vi "UI_visual2.vi"() -> ()   [LabVIEW 2017]
uses:
  <vilib>/Utility/miscctls.llb/LV3DPointTypeDef.ctl
  <vilib>/Analysis/coordinate.llb/Euler Rotation Order.ctl
  <vilib>/picture/3D Picture Control/Object/Create Object (drawable).vi
  <vilib>/picture/3D Picture Control/Object/Create Object (name).vi
  <vilib>/picture/3D Picture Control/Object/Add Object (no reference).vi
  <vilib>/picture/3D Picture Control/Helpers/Apply Texture (no reference).vi
  <vilib>/picture/3D Picture Control/NI_3D Picture Control.lvlib
  <vilib>/Analysis/NI_AALPro.lvlib
  <vilib>/picture/3D Picture Control/Helpers/Set Clip Plane (no reference).vi
panel:
  out "V_ini [m/s]":dbl[][](array[numeric])
  out "Euler Angles [rad]":dbl[](array[numeric])
  in  "Sim_Time":dbl=40.0
  in  "Tab Control":T1(tab)
  out "Position":dbl[][](graph)
  out "Velocity [m/s]":cluster{dbl, dbl, "V_ini [m/s]":dbl[]}(graph)
  out "Quaternions":dbl[][](graph)
  out "Euler Angles [º]":cluster{dbl, dbl, dbl[][]}(graph)
  out "Body Rates":dbl[][](graph)
  out "Body accelerations":dbl[][](graph)
  out "Malpha/Mbeta":dbl[][](graph)
  out "AoA":dbl[][](graph)
  out "TVA angles":dbl[][](graph)
  out "Oil Consumption":dbl[][](graph)
  out "Bending Moments":dbl[][](graph)
  out "Aerodynamic pressure":dbl[](graph)
  out "Sim_Stopped":bool
  in  "stop Host":bool
  in  "Run_SIM":bool
  out "time[s]":dbl
  out "Euler Angles [º]":dbl[](array[numeric])
  out "B-frame [m]":cluster{"X":sgl, "Y":sgl, "Z":sgl}
  in  "B-frame Translation 2":cluster{"X":sgl, "Y":sgl, "Z":sgl}
  in  "N-frame rot":dbl[](array[numeric])
  in  "Up Direction":T2={"X"=0.0, "Y"=0.0, "Z"=1.0}
  out "3D Picture Control":refnum<vi>(3d-picture)
  in  "error in (no error)":errorcluster
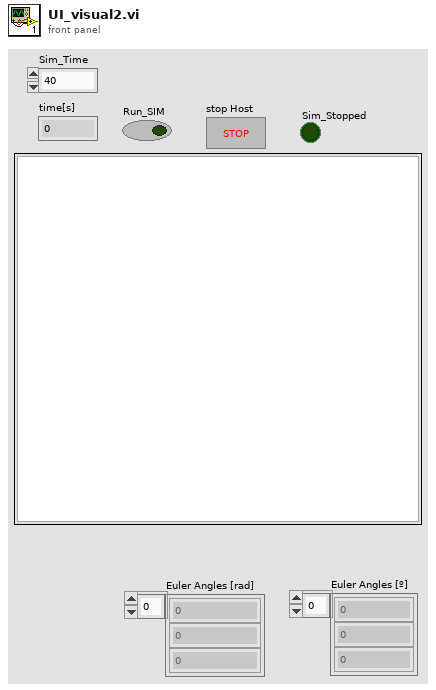
[diagram p1: front panel]
types:
  T1 = enum32{"Position", "Velocity", "Attitude Quaternions", "Attitude Euler Angles", "Body Rates", "Body Accel", "Malpha/ Mbeta", "AoA", "TVA nozzle angles", "Oil Consumption", "Bending Moments", "Aerodynamic pressure"}
  T2 = typedef "LV3DPointTypeDef.ctl" = cluster{"X":sgl, "Y":sgl, "Z":sgl}
  T3 = enum16{"As a Decal", "With Modulation", "With Blending", "As a replacement"}
  T4 = cluster{"Red":sgl, "Green":sgl, "Blue":sgl, "Alpha":sgl}
  T5 = typedef "NI_AALPro.lvlib/Euler Rotation Order.ctl" = u16
  T6 = typedef "imagedata.ctl" = cluster{"image type":i32, "image depth":i32, "image":u8[], "mask":u8[], "colors":u32[], "Rectangle":cluster{"left":i16, "top":i16, "right":i16, "bottom":i16}}
  T7 = cluster{"element":dbl, "element":dbl, "element":dbl}
  T8 = cluster{dbl, "latd_ini [º]":dbl, "lon_ini [º]":dbl, "alt_ini(m)":dbl, "V_ini [m/s]":dbl[], "q ini":dbl[], dbl[], "W ini [rad/s]":dbl[], "acc":dbl[], dbl[], dbl[], "TVA_b":dbl[], "array":dbl[], "array":dbl[], "Pdin":dbl}
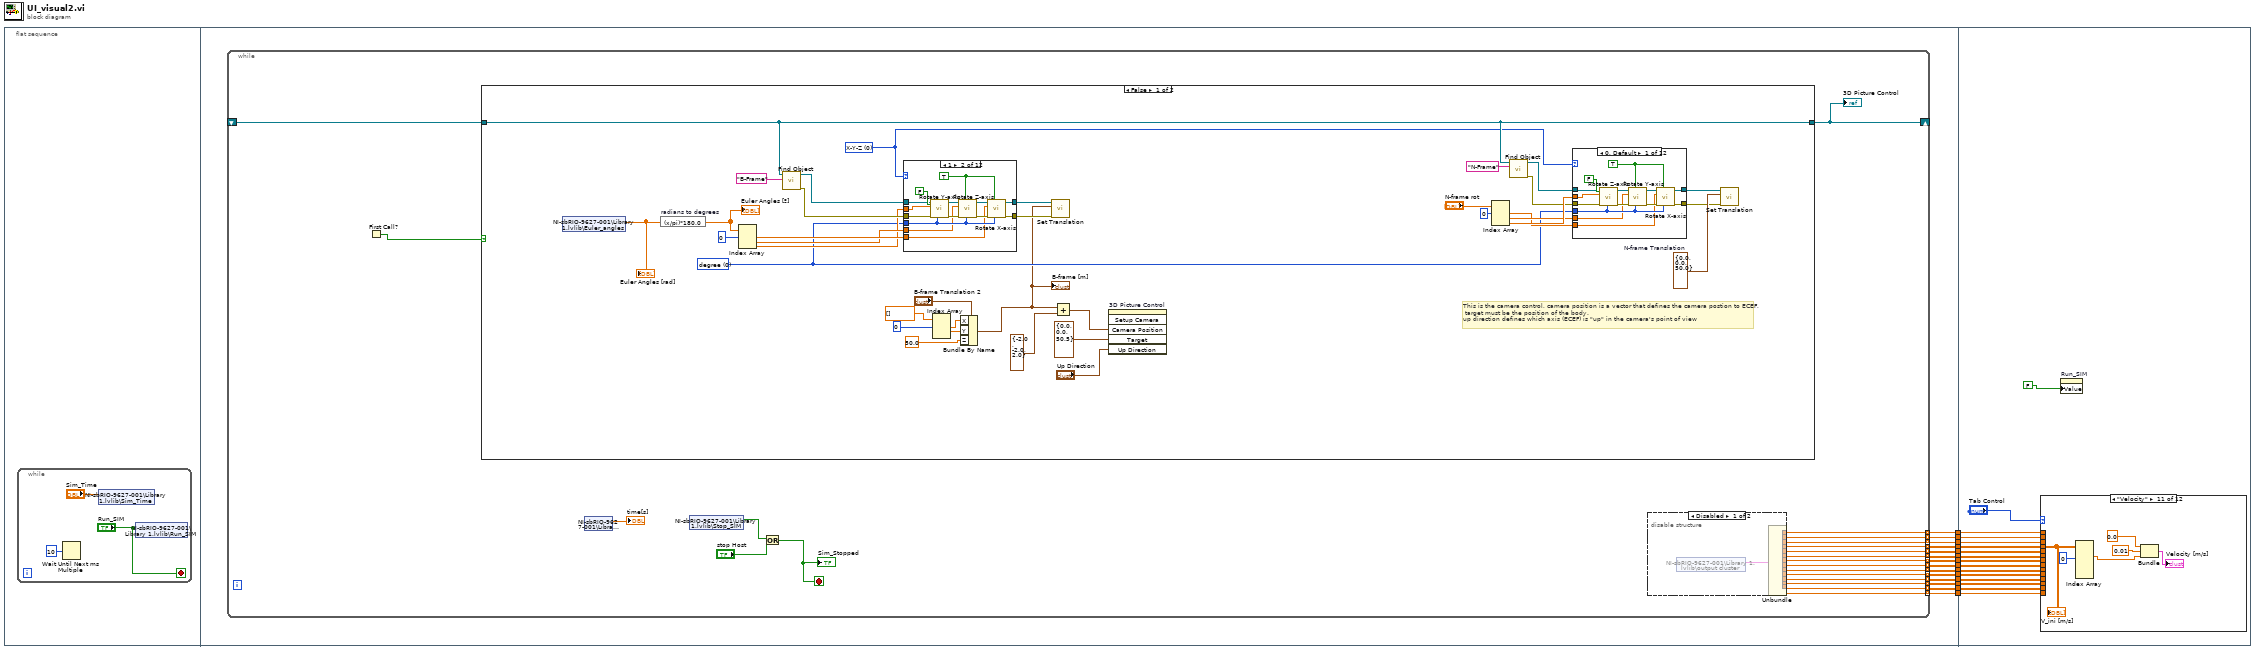
[diagram p0: block diagram]
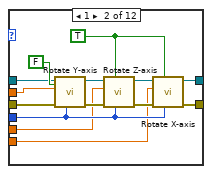
[diagram p3: hidden frame]
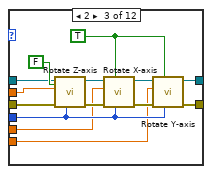
[diagram p4: hidden frame]
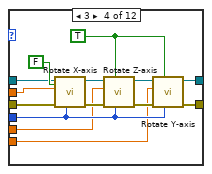
[diagram p5: hidden frame]
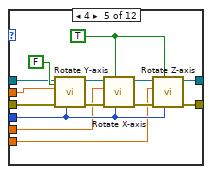
[diagram p6: hidden frame]
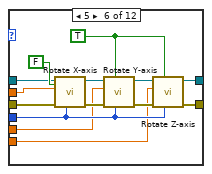
[diagram p7: hidden frame]
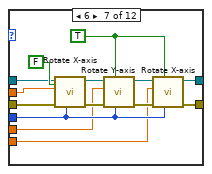
[diagram p8: hidden frame]
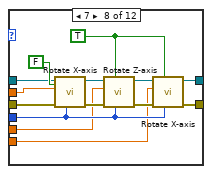
[diagram p9: hidden frame]
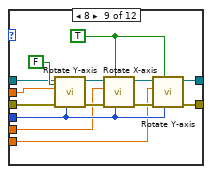
[diagram p10: hidden frame]
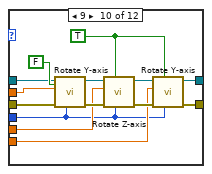
[diagram p11: hidden frame]
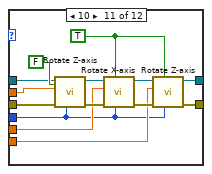
[diagram p12: hidden frame]
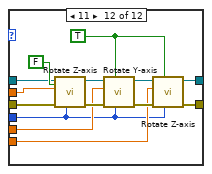
[diagram p13: hidden frame]
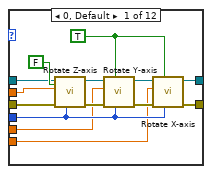
[diagram p14: hidden frame]
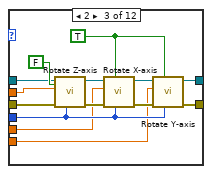
[diagram p15: hidden frame]
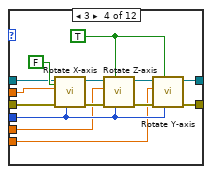
[diagram p16: hidden frame]
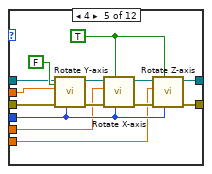
[diagram p17: hidden frame]
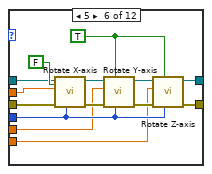
[diagram p18: hidden frame]
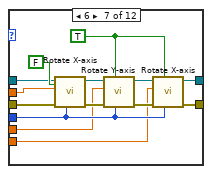
[diagram p19: hidden frame]
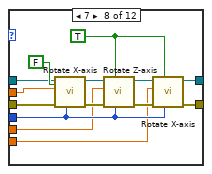
[diagram p20: hidden frame]
diagram:
  n1 = flat-sequence {
    tunnel: [w31] -> w14
    tunnel: [w30] -> w13
    tunnel: [w29] -> w12
    tunnel: [w28] -> w11
    tunnel: [w27] -> w10
    tunnel: [w26] -> w9
    tunnel: [w25] -> w8
    tunnel: [w24] -> w7
    tunnel: [w23] -> w6
    tunnel: [w22] -> w5
    tunnel: [w21] -> w4
    tunnel: [w20] -> w3
    tunnel: [w19] -> w2
    tunnel: [w18] -> w1
    tunnel: w14 -> [w533]
    tunnel: w13 -> [w532]
    tunnel: w12 -> [w531]
    tunnel: w11 -> [w530]
    tunnel: w10 -> [w529]
    tunnel: w9 -> [w528]
    tunnel: w8 -> [w527]
    tunnel: w7 -> [w526]
    tunnel: w6 -> [w525]
    tunnel: w5 -> [w524]
    tunnel: w4 -> [w523]
    tunnel: w3 -> [w522]
    tunnel: w2 -> [w521]
    tunnel: w1 -> [w520]
    frame #0 {
      n2 = while {
        stop <- "Run_SIM" stop-if-true
        n3 = Wait Until Next ms Multiple(millisecond multiple=u32 10) -> ()  [unwired: 1 out]
        n4 = shared-variable "NI-sbRIO-9627-001\\Library 1.lvlib\\Sim_Time"("Sim_Time") -> ()  [unwired: 1 in, 1 out]
        n5 = shared-variable "NI-sbRIO-9627-001\\Library 1.lvlib\\Run_SIM"("Run_SIM") -> ()  [unwired: 1 in, 1 out]
      }
    }
    frame #1 {
      n6 = while {
        shift-right: [w51] -> _
        shift-left: _ -> [w52]
        tunnel: [w45] -> w31 mode=indexing
        tunnel: [w44] -> w30 mode=indexing
        tunnel: [w43] -> w29 mode=indexing
        tunnel: [w42] -> w28 mode=indexing
        tunnel: [w41] -> w27 mode=indexing
        tunnel: [w40] -> w26 mode=indexing
        tunnel: [w39] -> w25 mode=indexing
        tunnel: [w38] -> w24 mode=indexing
        tunnel: [w37] -> w23 mode=indexing
        tunnel: [w36] -> w22 mode=indexing
        tunnel: [w35] -> w21 mode=indexing
        tunnel: [w34] -> w20 mode=indexing
        tunnel: [w33] -> w19 mode=indexing
        tunnel: [w32] -> w18 mode=indexing
        stop <- w48 stop-if-true
        n7 = First Call?() -> (First Call?: T/F=w50:bool)
        n8 = case shown="False" w50 {
          tunnel: [w84 w447] -> w51
          tunnel: w52 -> [w84 _]
          frame False {
            w83 = T5 0 items=["X-Y-Z", "X-Z-Y", "Y-X-Z", "Y-Z-X", "Z-X-Y", "Z-Y-X", "X-Y-X", "X-Z-X", "Y-X-Y", "Y-Z-Y", "Z-X-Z", "Z-Y-Z"] ("rotation order")
            w94 = cluster{"X":sgl, "Y":sgl, "Z":sgl} {"X"=0.0, "Y"=0.0, "Z"=50.0}  # N-frame Translation
            w82 = u16 0 items=["degree", "radians"] ("angle unit")
            # "This is the camera control, camera position is a vector that defines the camera postion to ECEF,\n target must be the position of the body. \nup direction defines which axis (ECEF) is \"up\" in the camera's point of view"
            n9 = shared-variable "NI-sbRIO-9627-001\\Library 1.lvlib\\Euler_angles"() -> (w76:dbl[])  [unwired: 1 in, 1 out]
            "Euler Angles [rad]" <- w76
            n10 = expression code="(x/pi)*180.0" "radians to degrees"(w76) -> (w77:dbl[])
            "Euler Angles [º]" <- w77
            n11 = Index Array(array=w77, index #1=0 ("index")) -> (element #1=w102:dbl, element #2=w99:dbl, element #3=w98:dbl)  [unwired: 2 in]
            n12 = call <vilib>:"Find Object.vi"("Object Name"="B-Frame", "Scene Refnum"=w84) -> ("error out"=w100:errorcluster, "Object Refnum"=w101:refnum<vi>)  [unwired: 8 in]
            n13 = case shown="1" w83 {
              tunnel: w102 -> [w276 w292 w306 w320 w330 w348 w362 w376 w390 w401 w415 w429]
              tunnel: w101 -> [w279 w289 w302 w316 w334 w344 w361 w375 w386 w405 w419 w433]
              tunnel: w100 -> [w278 w288 w303 w317 w333 w345 w360 w374 w387 w404 w418 w432]
              tunnel: w99 -> [w275 w290 w305 w319 w331 w347 w358 w372 w389 w402 w416 w431]
              tunnel: w98 -> [w274 w291 w304 w318 w332 w346 w359 w373 w388 w403 w417 w430]
              tunnel: w82 -> [w277 w293 w307 w321 w335 w349 w363 w377 w391 w400 w414 w428]
              tunnel: [w273 w287 w301 w315 w329 w343 w357 w371 w385 w399 w413 w427] -> w96
              tunnel: [w272 w286 w300 w314 w328 w342 w356 w370 w384 w398 w412 w426] -> w95
              frame 0, Default {
                w285 = TRUE ("Relative?")
                n14 = call <vilib>:"Rotate Z-axis.vi"("angle unit"=w277, "Relative?"=FALSE, "error in (no error)"=w278, "angle"=w274, "Scene Object In"=w279) -> ("error out"=w282:errorcluster, "Scene Object Out"=w283:refnum<vi>)  [unwired: 5 in]
                n15 = call <vilib>:"Rotate Y-axis.vi"("angle unit"=w277, "Relative?"=w285, "error in (no error)"=w282, "angle"=w275, "Scene Object In"=w283) -> ("error out"=w281:errorcluster, "Scene Object Out"=w280:refnum<vi>)  [unwired: 5 in]
                n16 = call <vilib>:"Rotate X-axis.vi"("angle unit"=w277, "Relative?"=w285, "error in (no error)"=w281, "angle"=w276, "Scene Object In"=w280) -> ("error out"=w272:errorcluster, "Scene Object Out"=w273:refnum<vi>)  [unwired: 5 in]
              }
              frame 1 {
                w296 = TRUE ("Relative?")
                n17 = call <vilib>:"Rotate Y-axis.vi"("angle unit"=w293, "Relative?"=FALSE, "error in (no error)"=w288, "angle"=w291, "Scene Object In"=w289) -> ("error out"=w297:errorcluster, "Scene Object Out"=w298:refnum<vi>)  [unwired: 5 in]
                n18 = call <vilib>:"Rotate Z-axis.vi"("angle unit"=w293, "Relative?"=w296, "error in (no error)"=w297, "angle"=w290, "Scene Object In"=w298) -> ("error out"=w294:errorcluster, "Scene Object Out"=w295:refnum<vi>)  [unwired: 5 in]
                n19 = call <vilib>:"Rotate X-axis.vi"("angle unit"=w293, "Relative?"=w296, "error in (no error)"=w294, "angle"=w292, "Scene Object In"=w295) -> ("error out"=w286:errorcluster, "Scene Object Out"=w287:refnum<vi>)  [unwired: 5 in]
              }
              frame 2 {
                w308 = TRUE ("Relative?")
                n20 = call <vilib>:"Rotate Z-axis.vi"("angle unit"=w307, "Relative?"=FALSE, "error in (no error)"=w303, "angle"=w304, "Scene Object In"=w302) -> ("error out"=w311:errorcluster, "Scene Object Out"=w312:refnum<vi>)  [unwired: 5 in]
                n21 = call <vilib>:"Rotate X-axis.vi"("angle unit"=w307, "Relative?"=w308, "error in (no error)"=w311, "angle"=w305, "Scene Object In"=w312) -> ("error out"=w309:errorcluster, "Scene Object Out"=w310:refnum<vi>)  [unwired: 5 in]
                n22 = call <vilib>:"Rotate Y-axis.vi"("angle unit"=w307, "Relative?"=w308, "error in (no error)"=w309, "angle"=w306, "Scene Object In"=w310) -> ("error out"=w300:errorcluster, "Scene Object Out"=w301:refnum<vi>)  [unwired: 5 in]
              }
              frame 3 {
                w326 = TRUE ("Relative?")
                n23 = call <vilib>:"Rotate X-axis.vi"("angle unit"=w321, "Relative?"=FALSE, "error in (no error)"=w317, "angle"=w318, "Scene Object In"=w316) -> ("error out"=w324:errorcluster, "Scene Object Out"=w325:refnum<vi>)  [unwired: 5 in]
                n24 = call <vilib>:"Rotate Z-axis.vi"("angle unit"=w321, "Relative?"=w326, "error in (no error)"=w324, "angle"=w319, "Scene Object In"=w325) -> ("error out"=w322:errorcluster, "Scene Object Out"=w323:refnum<vi>)  [unwired: 5 in]
                n25 = call <vilib>:"Rotate Y-axis.vi"("angle unit"=w321, "Relative?"=w326, "error in (no error)"=w322, "angle"=w320, "Scene Object In"=w323) -> ("error out"=w314:errorcluster, "Scene Object Out"=w315:refnum<vi>)  [unwired: 5 in]
              }
              frame 4 {
                w340 = TRUE ("Relative?")
                n26 = call <vilib>:"Rotate Y-axis.vi"("angle unit"=w335, "Relative?"=FALSE, "error in (no error)"=w333, "angle"=w332, "Scene Object In"=w334) -> ("error out"=w336:errorcluster, "Scene Object Out"=w337:refnum<vi>)  [unwired: 5 in]
                n27 = call <vilib>:"Rotate X-axis.vi"("angle unit"=w335, "Relative?"=w340, "error in (no error)"=w336, "angle"=w331, "Scene Object In"=w337) -> ("error out"=w339:errorcluster, "Scene Object Out"=w338:refnum<vi>)  [unwired: 5 in]
                n28 = call <vilib>:"Rotate Z-axis.vi"("angle unit"=w335, "Relative?"=w340, "error in (no error)"=w339, "angle"=w330, "Scene Object In"=w338) -> ("error out"=w328:errorcluster, "Scene Object Out"=w329:refnum<vi>)  [unwired: 5 in]
              }
              frame 5 {
                w353 = TRUE ("Relative?")
                n29 = call <vilib>:"Rotate X-axis.vi"("angle unit"=w349, "Relative?"=FALSE, "error in (no error)"=w345, "angle"=w346, "Scene Object In"=w344) -> ("error out"=w351:errorcluster, "Scene Object Out"=w352:refnum<vi>)  [unwired: 5 in]
                n30 = call <vilib>:"Rotate Y-axis.vi"("angle unit"=w349, "Relative?"=w353, "error in (no error)"=w351, "angle"=w347, "Scene Object In"=w352) -> ("error out"=w355:errorcluster, "Scene Object Out"=w354:refnum<vi>)  [unwired: 5 in]
                n31 = call <vilib>:"Rotate Z-axis.vi"("angle unit"=w349, "Relative?"=w353, "error in (no error)"=w355, "angle"=w348, "Scene Object In"=w354) -> ("error out"=w342:errorcluster, "Scene Object Out"=w343:refnum<vi>)  [unwired: 5 in]
              }
              frame 6 {
                w366 = TRUE ("Relative?")
                n32 = call <vilib>:"Rotate X-axis.vi"("angle unit"=w363, "Relative?"=FALSE, "error in (no error)"=w360, "angle"=w359, "Scene Object In"=w361) -> ("error out"=w368:errorcluster, "Scene Object Out"=w369:refnum<vi>)  [unwired: 5 in]
                n33 = call <vilib>:"Rotate Y-axis.vi"("angle unit"=w363, "Relative?"=w366, "error in (no error)"=w368, "angle"=w358, "Scene Object In"=w369) -> ("error out"=w364:errorcluster, "Scene Object Out"=w365:refnum<vi>)  [unwired: 5 in]
                n34 = call <vilib>:"Rotate X-axis.vi"("angle unit"=w363, "Relative?"=w366, "error in (no error)"=w364, "angle"=w362, "Scene Object In"=w365) -> ("error out"=w356:errorcluster, "Scene Object Out"=w357:refnum<vi>)  [unwired: 5 in]
              }
              frame 7 {
                w382 = TRUE ("Relative?")
                n35 = call <vilib>:"Rotate X-axis.vi"("angle unit"=w377, "Relative?"=FALSE, "error in (no error)"=w374, "angle"=w373, "Scene Object In"=w375) -> ("error out"=w380:errorcluster, "Scene Object Out"=w381:refnum<vi>)  [unwired: 5 in]
                n36 = call <vilib>:"Rotate Z-axis.vi"("angle unit"=w377, "Relative?"=w382, "error in (no error)"=w380, "angle"=w372, "Scene Object In"=w381) -> ("error out"=w379:errorcluster, "Scene Object Out"=w378:refnum<vi>)  [unwired: 5 in]
                n37 = call <vilib>:"Rotate X-axis.vi"("angle unit"=w377, "Relative?"=w382, "error in (no error)"=w379, "angle"=w376, "Scene Object In"=w378) -> ("error out"=w370:errorcluster, "Scene Object Out"=w371:refnum<vi>)  [unwired: 5 in]
              }
              frame 8 {
                w396 = TRUE ("Relative?")
                n38 = call <vilib>:"Rotate Y-axis.vi"("angle unit"=w391, "Relative?"=FALSE, "error in (no error)"=w387, "angle"=w388, "Scene Object In"=w386) -> ("error out"=w394:errorcluster, "Scene Object Out"=w395:refnum<vi>)  [unwired: 5 in]
                n39 = call <vilib>:"Rotate X-axis.vi"("angle unit"=w391, "Relative?"=w396, "error in (no error)"=w394, "angle"=w389, "Scene Object In"=w395) -> ("error out"=w393:errorcluster, "Scene Object Out"=w392:refnum<vi>)  [unwired: 5 in]
                n40 = call <vilib>:"Rotate Y-axis.vi"("angle unit"=w391, "Relative?"=w396, "error in (no error)"=w393, "angle"=w390, "Scene Object In"=w392) -> ("error out"=w384:errorcluster, "Scene Object Out"=w385:refnum<vi>)  [unwired: 5 in]
              }
              frame 9 {
                w410 = TRUE ("Relative?")
                n41 = call <vilib>:"Rotate Y-axis.vi"("angle unit"=w400, "Relative?"=FALSE, "error in (no error)"=w404, "angle"=w403, "Scene Object In"=w405) -> ("error out"=w408:errorcluster, "Scene Object Out"=w409:refnum<vi>)  [unwired: 5 in]
                n42 = call <vilib>:"Rotate Z-axis.vi"("angle unit"=w400, "Relative?"=w410, "error in (no error)"=w408, "angle"=w402, "Scene Object In"=w409) -> ("error out"=w407:errorcluster, "Scene Object Out"=w406:refnum<vi>)  [unwired: 5 in]
                n43 = call <vilib>:"Rotate Y-axis.vi"("angle unit"=w400, "Relative?"=w410, "error in (no error)"=w407, "angle"=w401, "Scene Object In"=w406) -> ("error out"=w398:errorcluster, "Scene Object Out"=w399:refnum<vi>)  [unwired: 5 in]
              }
              frame 10 {
                w424 = TRUE ("Relative?")
                n44 = call <vilib>:"Rotate Z-axis.vi"("angle unit"=w414, "Relative?"=FALSE, "error in (no error)"=w418, "angle"=w417, "Scene Object In"=w419) -> ("error out"=w422:errorcluster, "Scene Object Out"=w423:refnum<vi>)  [unwired: 5 in]
                n45 = call <vilib>:"Rotate X-axis.vi"("angle unit"=w414, "Relative?"=w424, "error in (no error)"=w422, "angle"=w416, "Scene Object In"=w423) -> ("error out"=w421:errorcluster, "Scene Object Out"=w420:refnum<vi>)  [unwired: 5 in]
                n46 = call <vilib>:"Rotate Z-axis.vi"("angle unit"=w414, "Relative?"=w424, "error in (no error)"=w421, "angle"=w415, "Scene Object In"=w420) -> ("error out"=w412:errorcluster, "Scene Object Out"=w413:refnum<vi>)  [unwired: 5 in]
              }
              frame 11 {
                w438 = TRUE ("Relative?")
                n47 = call <vilib>:"Rotate Z-axis.vi"("angle unit"=w428, "Relative?"=FALSE, "error in (no error)"=w432, "angle"=w430, "Scene Object In"=w433) -> ("error out"=w436:errorcluster, "Scene Object Out"=w437:refnum<vi>)  [unwired: 5 in]
                n48 = call <vilib>:"Rotate Y-axis.vi"("angle unit"=w428, "Relative?"=w438, "error in (no error)"=w436, "angle"=w431, "Scene Object In"=w437) -> ("error out"=w435:errorcluster, "Scene Object Out"=w434:refnum<vi>)  [unwired: 5 in]
                n49 = call <vilib>:"Rotate Z-axis.vi"("angle unit"=w428, "Relative?"=w438, "error in (no error)"=w435, "angle"=w429, "Scene Object In"=w434) -> ("error out"=w426:errorcluster, "Scene Object Out"=w427:refnum<vi>)  [unwired: 5 in]
              }
            }
            n50 = Index Array(array=dbl[] [], index #1=0 ("index")) -> (element #1=w79:dbl, element #2=w78:dbl)  [unwired: 2 in, 1 out]
            n51 = Bundle By Name(cluster="B-frame Translation 2", "X"=w79, "Y"=w78, "Z"=50.0 ("Double")) -> (w70:cluster{"X":sgl, "Y":sgl, "Z":sgl})
            "B-frame [m]" <- w70
            n52 = call <vilib>:"Set Translation.vi"("error in (no error)"=w95, "Translation"=w70, "Scene Object"=w96) -> ()  [unwired: 7 in, 2 out]
            n53 = Add(x=w70, y=T2 {"X"=-2.0, "Y"=-2.0, "Z"=2.0} ("Camera Position control")) -> (x+y=w71:T2)
            n54 = invoke on="3D Picture Control" class="SceneGraphDisp (strict)" method="Setup Camera"("Camera Position"=w71, "Target"=T2 {"X"=0.0, "Y"=0.0, "Z"=50.5}, "Up Direction"="Up Direction") -> ()  [unwired: 3 in, 6 out]
            n55 = Index Array(array="N-frame rot", index #1=0 ("index")) -> (element #1=w86:dbl, element #2=w89:dbl, element #3=w90:dbl)  [unwired: 2 in]
            n56 = call <vilib>:"Find Object.vi"("Object Name"="N-Frame", "Scene Refnum"=w84) -> ("error out"=w88:errorcluster, "Object Refnum"=w87:refnum<vi>)  [unwired: 8 in]
            n57 = case shown="0, Default" w83 {
              tunnel: w86 -> [w108 w124 w138 w152 w162 w180 w194 w208 w222 w233 w247 w261]
              tunnel: w87 -> [w111 w121 w134 w148 w166 w176 w193 w207 w218 w237 w251 w265]
              tunnel: w88 -> [w110 w120 w135 w149 w165 w177 w192 w206 w219 w236 w250 w264]
              tunnel: w89 -> [w107 w122 w137 w151 w163 w179 w190 w204 w221 w234 w248 w263]
              tunnel: w90 -> [w106 w123 w136 w150 w164 w178 w191 w205 w220 w235 w249 w262]
              tunnel: w82 -> [w109 w125 w139 w153 w167 w181 w195 w209 w223 w232 w246 w260]
              tunnel: [w105 w119 w133 w147 w161 w175 w189 w203 w217 w231 w245 w259] -> w92
              tunnel: [w104 w118 w132 w146 w160 w174 w188 w202 w216 w230 w244 w258] -> w93
              frame 0, Default {
                w117 = TRUE ("Relative?")
                n58 = call <vilib>:"Rotate Z-axis.vi"("angle unit"=w109, "Relative?"=FALSE, "error in (no error)"=w110, "angle"=w106, "Scene Object In"=w111) -> ("error out"=w114:errorcluster, "Scene Object Out"=w115:refnum<vi>)  [unwired: 5 in]
                n59 = call <vilib>:"Rotate Y-axis.vi"("angle unit"=w109, "Relative?"=w117, "error in (no error)"=w114, "angle"=w107, "Scene Object In"=w115) -> ("error out"=w113:errorcluster, "Scene Object Out"=w112:refnum<vi>)  [unwired: 5 in]
                n60 = call <vilib>:"Rotate X-axis.vi"("angle unit"=w109, "Relative?"=w117, "error in (no error)"=w113, "angle"=w108, "Scene Object In"=w112) -> ("error out"=w104:errorcluster, "Scene Object Out"=w105:refnum<vi>)  [unwired: 5 in]
              }
              frame 1 {
                w128 = TRUE ("Relative?")
                n61 = call <vilib>:"Rotate Y-axis.vi"("angle unit"=w125, "Relative?"=FALSE, "error in (no error)"=w120, "angle"=w123, "Scene Object In"=w121) -> ("error out"=w129:errorcluster, "Scene Object Out"=w130:refnum<vi>)  [unwired: 5 in]
                n62 = call <vilib>:"Rotate Z-axis.vi"("angle unit"=w125, "Relative?"=w128, "error in (no error)"=w129, "angle"=w122, "Scene Object In"=w130) -> ("error out"=w126:errorcluster, "Scene Object Out"=w127:refnum<vi>)  [unwired: 5 in]
                n63 = call <vilib>:"Rotate X-axis.vi"("angle unit"=w125, "Relative?"=w128, "error in (no error)"=w126, "angle"=w124, "Scene Object In"=w127) -> ("error out"=w118:errorcluster, "Scene Object Out"=w119:refnum<vi>)  [unwired: 5 in]
              }
              frame 2 {
                w140 = TRUE ("Relative?")
                n64 = call <vilib>:"Rotate Z-axis.vi"("angle unit"=w139, "Relative?"=FALSE, "error in (no error)"=w135, "angle"=w136, "Scene Object In"=w134) -> ("error out"=w143:errorcluster, "Scene Object Out"=w144:refnum<vi>)  [unwired: 5 in]
                n65 = call <vilib>:"Rotate X-axis.vi"("angle unit"=w139, "Relative?"=w140, "error in (no error)"=w143, "angle"=w137, "Scene Object In"=w144) -> ("error out"=w141:errorcluster, "Scene Object Out"=w142:refnum<vi>)  [unwired: 5 in]
                n66 = call <vilib>:"Rotate Y-axis.vi"("angle unit"=w139, "Relative?"=w140, "error in (no error)"=w141, "angle"=w138, "Scene Object In"=w142) -> ("error out"=w132:errorcluster, "Scene Object Out"=w133:refnum<vi>)  [unwired: 5 in]
              }
              frame 3 {
                w158 = TRUE ("Relative?")
                n67 = call <vilib>:"Rotate X-axis.vi"("angle unit"=w153, "Relative?"=FALSE, "error in (no error)"=w149, "angle"=w150, "Scene Object In"=w148) -> ("error out"=w156:errorcluster, "Scene Object Out"=w157:refnum<vi>)  [unwired: 5 in]
                n68 = call <vilib>:"Rotate Z-axis.vi"("angle unit"=w153, "Relative?"=w158, "error in (no error)"=w156, "angle"=w151, "Scene Object In"=w157) -> ("error out"=w154:errorcluster, "Scene Object Out"=w155:refnum<vi>)  [unwired: 5 in]
                n69 = call <vilib>:"Rotate Y-axis.vi"("angle unit"=w153, "Relative?"=w158, "error in (no error)"=w154, "angle"=w152, "Scene Object In"=w155) -> ("error out"=w146:errorcluster, "Scene Object Out"=w147:refnum<vi>)  [unwired: 5 in]
              }
              frame 4 {
                w172 = TRUE ("Relative?")
                n70 = call <vilib>:"Rotate Y-axis.vi"("angle unit"=w167, "Relative?"=FALSE, "error in (no error)"=w165, "angle"=w164, "Scene Object In"=w166) -> ("error out"=w168:errorcluster, "Scene Object Out"=w169:refnum<vi>)  [unwired: 5 in]
                n71 = call <vilib>:"Rotate X-axis.vi"("angle unit"=w167, "Relative?"=w172, "error in (no error)"=w168, "angle"=w163, "Scene Object In"=w169) -> ("error out"=w171:errorcluster, "Scene Object Out"=w170:refnum<vi>)  [unwired: 5 in]
                n72 = call <vilib>:"Rotate Z-axis.vi"("angle unit"=w167, "Relative?"=w172, "error in (no error)"=w171, "angle"=w162, "Scene Object In"=w170) -> ("error out"=w160:errorcluster, "Scene Object Out"=w161:refnum<vi>)  [unwired: 5 in]
              }
              frame 5 {
                w185 = TRUE ("Relative?")
                n73 = call <vilib>:"Rotate X-axis.vi"("angle unit"=w181, "Relative?"=FALSE, "error in (no error)"=w177, "angle"=w178, "Scene Object In"=w176) -> ("error out"=w183:errorcluster, "Scene Object Out"=w184:refnum<vi>)  [unwired: 5 in]
                n74 = call <vilib>:"Rotate Y-axis.vi"("angle unit"=w181, "Relative?"=w185, "error in (no error)"=w183, "angle"=w179, "Scene Object In"=w184) -> ("error out"=w187:errorcluster, "Scene Object Out"=w186:refnum<vi>)  [unwired: 5 in]
                n75 = call <vilib>:"Rotate Z-axis.vi"("angle unit"=w181, "Relative?"=w185, "error in (no error)"=w187, "angle"=w180, "Scene Object In"=w186) -> ("error out"=w174:errorcluster, "Scene Object Out"=w175:refnum<vi>)  [unwired: 5 in]
              }
              frame 6 {
                w198 = TRUE ("Relative?")
                n76 = call <vilib>:"Rotate X-axis.vi"("angle unit"=w195, "Relative?"=FALSE, "error in (no error)"=w192, "angle"=w191, "Scene Object In"=w193) -> ("error out"=w200:errorcluster, "Scene Object Out"=w201:refnum<vi>)  [unwired: 5 in]
                n77 = call <vilib>:"Rotate Y-axis.vi"("angle unit"=w195, "Relative?"=w198, "error in (no error)"=w200, "angle"=w190, "Scene Object In"=w201) -> ("error out"=w196:errorcluster, "Scene Object Out"=w197:refnum<vi>)  [unwired: 5 in]
                n78 = call <vilib>:"Rotate X-axis.vi"("angle unit"=w195, "Relative?"=w198, "error in (no error)"=w196, "angle"=w194, "Scene Object In"=w197) -> ("error out"=w188:errorcluster, "Scene Object Out"=w189:refnum<vi>)  [unwired: 5 in]
              }
              frame 7 {
                w214 = TRUE ("Relative?")
                n79 = call <vilib>:"Rotate X-axis.vi"("angle unit"=w209, "Relative?"=FALSE, "error in (no error)"=w206, "angle"=w205, "Scene Object In"=w207) -> ("error out"=w212:errorcluster, "Scene Object Out"=w213:refnum<vi>)  [unwired: 5 in]
                n80 = call <vilib>:"Rotate Z-axis.vi"("angle unit"=w209, "Relative?"=w214, "error in (no error)"=w212, "angle"=w204, "Scene Object In"=w213) -> ("error out"=w211:errorcluster, "Scene Object Out"=w210:refnum<vi>)  [unwired: 5 in]
                n81 = call <vilib>:"Rotate X-axis.vi"("angle unit"=w209, "Relative?"=w214, "error in (no error)"=w211, "angle"=w208, "Scene Object In"=w210) -> ("error out"=w202:errorcluster, "Scene Object Out"=w203:refnum<vi>)  [unwired: 5 in]
              }
              frame 8 {
                w228 = TRUE ("Relative?")
                n82 = call <vilib>:"Rotate Y-axis.vi"("angle unit"=w223, "Relative?"=FALSE, "error in (no error)"=w219, "angle"=w220, "Scene Object In"=w218) -> ("error out"=w226:errorcluster, "Scene Object Out"=w227:refnum<vi>)  [unwired: 5 in]
                n83 = call <vilib>:"Rotate X-axis.vi"("angle unit"=w223, "Relative?"=w228, "error in (no error)"=w226, "angle"=w221, "Scene Object In"=w227) -> ("error out"=w225:errorcluster, "Scene Object Out"=w224:refnum<vi>)  [unwired: 5 in]
                n84 = call <vilib>:"Rotate Y-axis.vi"("angle unit"=w223, "Relative?"=w228, "error in (no error)"=w225, "angle"=w222, "Scene Object In"=w224) -> ("error out"=w216:errorcluster, "Scene Object Out"=w217:refnum<vi>)  [unwired: 5 in]
              }
              frame 9 {
                w242 = TRUE ("Relative?")
                n85 = call <vilib>:"Rotate Y-axis.vi"("angle unit"=w232, "Relative?"=FALSE, "error in (no error)"=w236, "angle"=w235, "Scene Object In"=w237) -> ("error out"=w240:errorcluster, "Scene Object Out"=w241:refnum<vi>)  [unwired: 5 in]
                n86 = call <vilib>:"Rotate Z-axis.vi"("angle unit"=w232, "Relative?"=w242, "error in (no error)"=w240, "angle"=w234, "Scene Object In"=w241) -> ("error out"=w239:errorcluster, "Scene Object Out"=w238:refnum<vi>)  [unwired: 5 in]
                n87 = call <vilib>:"Rotate Y-axis.vi"("angle unit"=w232, "Relative?"=w242, "error in (no error)"=w239, "angle"=w233, "Scene Object In"=w238) -> ("error out"=w230:errorcluster, "Scene Object Out"=w231:refnum<vi>)  [unwired: 5 in]
              }
              frame 10 {
                w256 = TRUE ("Relative?")
                n88 = call <vilib>:"Rotate Z-axis.vi"("angle unit"=w246, "Relative?"=FALSE, "error in (no error)"=w250, "angle"=w249, "Scene Object In"=w251) -> ("error out"=w254:errorcluster, "Scene Object Out"=w255:refnum<vi>)  [unwired: 5 in]
                n89 = call <vilib>:"Rotate X-axis.vi"("angle unit"=w246, "Relative?"=w256, "error in (no error)"=w254, "angle"=w248, "Scene Object In"=w255) -> ("error out"=w253:errorcluster, "Scene Object Out"=w252:refnum<vi>)  [unwired: 5 in]
                n90 = call <vilib>:"Rotate Z-axis.vi"("angle unit"=w246, "Relative?"=w256, "error in (no error)"=w253, "angle"=w247, "Scene Object In"=w252) -> ("error out"=w244:errorcluster, "Scene Object Out"=w245:refnum<vi>)  [unwired: 5 in]
              }
              frame 11 {
                w270 = TRUE ("Relative?")
                n91 = call <vilib>:"Rotate Z-axis.vi"("angle unit"=w260, "Relative?"=FALSE, "error in (no error)"=w264, "angle"=w262, "Scene Object In"=w265) -> ("error out"=w268:errorcluster, "Scene Object Out"=w269:refnum<vi>)  [unwired: 5 in]
                n92 = call <vilib>:"Rotate Y-axis.vi"("angle unit"=w260, "Relative?"=w270, "error in (no error)"=w268, "angle"=w263, "Scene Object In"=w269) -> ("error out"=w267:errorcluster, "Scene Object Out"=w266:refnum<vi>)  [unwired: 5 in]
                n93 = call <vilib>:"Rotate Z-axis.vi"("angle unit"=w260, "Relative?"=w270, "error in (no error)"=w267, "angle"=w261, "Scene Object In"=w266) -> ("error out"=w258:errorcluster, "Scene Object Out"=w259:refnum<vi>)  [unwired: 5 in]
              }
            }
            n94 = call <vilib>:"Set Translation.vi"("error in (no error)"=w93, "Translation"=w94, "Scene Object"=w92) -> ()  [unwired: 7 in, 2 out]
          }
          frame True {
            w441 = -50.0 ("element")
            w493 = 100 ("dimension size")
            (unwired) "world32k.bmp" ("name or relative path")
            w495 = sgl 1.0 ("Row Interval")
            # "Initial P ECEF"
            # "Branco"
            # "Cria o frame do corpo"
            # "Cria o frame de navegação"
            # "This loads the texture map and\nreadies it to use on the ground."
            # "Use the random height matrix\nto generate a height grid."
            n95 = disable-structure shown="Disabled" {
              disable-tunnel: [w499 _] -> w487
              disable-tunnel: [w498 _] -> w479
              frame Disabled {
                n96 = Strip Path(path=path "world32k.bmp") -> (stripped path=w496:path)  [unwired: 1 out]
                n97 = call <vilib>:"Read PNG File.vi"("path to PNG file"=w496) -> ("error out"=w498:errorcluster, "image data"=w499:T6)  [unwired: 1 in, 8 out]
              }
              frame Enabled {
              }
            }
            n98 = Initialize Array(0.0 ("element"), w493, w493) -> (w491:dbl[][])
            n99 = call <vilib>:"Create Height Field.vi"("Column Interval"=w495, "Row Interval"=w495, "Data"=w491) -> ("error out"=w477:errorcluster, "New Height Field Refnum"=w486:refnum<vi>)  [unwired: 1 in, 6 out]
            n100 = call-poly <vilib>:"Create Object.vi"("error in (no error)"=w477, "Geometry"=w486, "Name"="Base") -> ("error out"=w478:errorcluster, "Scene:New Object"=w488:refnum<vi>)  [unwired: 7 in]
            n101 = Merge Errors(w478, w479) -> (w442:errorcluster)
            n102 = call-poly <vilib>:"Apply Texture.vi"("Horizontal Wrap Mode"=enum16{"Clamp", "Repeat"}."Repeat", "error in (no error)"=w442, "Apply Mode"=T3."As a Decal", "Image Data"=w487, "Scene Object In"=w488) -> ("error out"=w480:errorcluster, "Scene Object Out"=w490:refnum<vi>)  [unwired: 5 in]
            n103 = Bundle("element"=w441, "element"=w441, "element"=50.0) -> (w494:T7)  [unwired: 1 out]
            n104 = call <vilib>:"Set Translation.vi"("error in (no error)"=w480, "Translation"=w494, "Scene Object"=w490) -> ("error out"=w481:errorcluster, "Translated Object"=w484:refnum<vi>)  [unwired: 7 out]
            n105 = call-poly <vilib>:"Create Object.vi"("error in (no error)"="error in (no error)", "Name"="world") -> ("error out"=w482:errorcluster, "Scene:New Object"=w483:refnum<vi>)  [unwired: 8 in]
            n106 = disable-structure shown="Disabled" {
              disable-tunnel: w484 -> [w517 _]
              disable-tunnel: w483 -> [w516 w518]
              disable-tunnel: w482 -> [w515 w519]
              disable-tunnel: w481 -> [w513 _]
              disable-tunnel: [w501 w519] -> w460
              disable-tunnel: [w500 w518] -> w459
              frame Disabled {
                w512 = sgl 0.0 ("A")
                # "Underneath Clipping\nPlane: z = 0"
                n107 = Merge Errors(w515, w513) -> (w514:errorcluster)
                n108 = call-poly <vilib>:"Add Object.vi"("error in (no error)"=w514, "New Object In"=w517, "Scene Object In"=w516) -> ("error out"=w502:errorcluster, "Scene Object Out"=w503:refnum<vi>)  [unwired: 7 in]
                n109 = Bundle By Name(cluster=cluster{"A":sgl, "B":sgl, "C":sgl, "D":sgl} {"A"=0.0, "B"=0.0, "C"=0.0, "D"=0.0} ("Plane"), "A"=w512, "B"=w512, "C"=sgl 1.0 ("B"), "D"=sgl 0.01 ("B")) -> (w509:cluster{"A":sgl, "B":sgl, "C":sgl, "D":sgl})
                n110 = call <vilib>:"Create Clip Plane.vi"("error in (no error)"=w502, "Number"=0, "Plane"=w509) -> ("error out"=w505:errorcluster, "New Clip Plane Refnum"=w507:refnum<vi>)  [unwired: 7 out]
                n111 = call-poly <vilib>:"Set Clip Plane.vi"("error in (no error)"=w505, "Clip Plane State"=enum16{"Inherit Value", "Off", "On"}."Off", "Clip Plane Refnum In"=w507, "Scene Object In"=w503) -> ("error out"=w501:errorcluster, "Scene Object Out"=w500:refnum<vi>)  [unwired: 6 in]
              }
              frame Enabled {
              }
            }
            n112 = call <vilib>:"Create 3D Axis.vi"("Axis label?"=TRUE, "Color"=T4 {"Red"=1.0, "Green"=1.0, "Blue"=1.0, "Alpha"=1.0}, "Length"=sgl 1.0 ("Radius"), "Name"="N-Frame") -> ("error out"=w452:errorcluster, "New Object Refnum"=w451:refnum<vi>)  [unwired: 6 in]
            n113 = call <vilib>:"Create 3D Axis.vi"("Axis label?"=TRUE, "Color"=T4 {"Red"=0.0, "Green"=1.0, "Blue"=0.0, "Alpha"=1.0}, "Length"=sgl 1.0 ("Radius"), "Name"="B-Frame") -> ("error out"=w461:errorcluster, "New Object Refnum"=w462:refnum<vi>)  [unwired: 6 in]
            n114 = call-poly <vilib>:"Create Object.vi"("Name"="Corpo") -> ("error out"=w455:errorcluster, "Scene:New Object"=w456:refnum<vi>)  [unwired: 9 in]
            n115 = call <vilib>:"Set Translation.vi"("error in (no error)"=w455, "Translation"=cluster{"X":sgl, "Y":sgl, "Z":sgl} {"X"=0.0, "Y"=0.0, "Z"=0.0}, "Scene Object"=w456) -> ("error out"=w458:errorcluster, "Translated Object"=w457:refnum<vi>)  [unwired: 7 out]
            n116 = Merge Errors(w458, w461) -> (w465:errorcluster)
            n117 = call-poly <vilib>:"Add Object.vi"("error in (no error)"=w465, "New Object In"=w462, "Scene Object In"=w457) -> ("error out"=w463:errorcluster, "Scene Object Out"=w464:refnum<vi>)  [unwired: 7 in]
            n118 = call <vilib>:"Set Translation.vi"("error in (no error)"=w452, "Translation"=cluster{"X":sgl, "Y":sgl, "Z":sgl} {"X"=0.0, "Y"=0.0, "Z"=0.0}, "Scene Object"=w451) -> ("error out"=w450:errorcluster, "Translated Object"=w449:refnum<vi>)  [unwired: 7 out]
            n119 = Merge Errors(w460, w463) -> (w475:errorcluster)
            n120 = call-poly <vilib>:"Add Object.vi"("error in (no error)"=w475, "New Object In"=w464, "Scene Object In"=w459) -> ("error out"=w469:errorcluster, "Scene Object Out"=w472:refnum<vi>)  [unwired: 7 in]
            n121 = Merge Errors(w469, w450) -> (w468:errorcluster)
            n122 = call-poly <vilib>:"Add Object.vi"("error in (no error)"=w468, "New Object In"=w449, "Scene Object In"=w472) -> ("Scene Object Out"=w447:refnum<vi>)  [unwired: 7 in, 1 out]
          }
        }
        "3D Picture Control" <- w51
        n123 = shared-variable "NI-sbRIO-9627-001\\Library 1.lvlib\\t"() -> (→"time[s]":dbl)  [unwired: 1 in, 1 out]
        n124 = shared-variable "NI-sbRIO-9627-001\\Library 1.lvlib\\Stop_SIM"() -> (w49:bool)  [unwired: 1 in, 1 out]
        n125 = Or(x=w49, y="stop Host") -> (x .or. y?=w48:bool)
        "Sim_Stopped" <- w48
        n126 = disable-structure shown="Disabled" {
          disable-tunnel: [w66 _] -> w45
          disable-tunnel: [w65 _] -> w44
          disable-tunnel: [w64 _] -> w43
          disable-tunnel: [w63 _] -> w42
          disable-tunnel: [w62 _] -> w41
          disable-tunnel: [w61 _] -> w40
          disable-tunnel: [w60 _] -> w39
          disable-tunnel: [w59 _] -> w38
          disable-tunnel: [w58 _] -> w37
          disable-tunnel: [w57 _] -> w36
          disable-tunnel: [w56 _] -> w35
          disable-tunnel: [w55 _] -> w34
          disable-tunnel: [w54 _] -> w33
          disable-tunnel: [w53 _] -> w32
          frame Disabled {
            n127 = shared-variable "NI-sbRIO-9627-001\\Library 1.lvlib\\output cluster"() -> (w67:T8)  [unwired: 1 in, 1 out]
            n128 = Unbundle(w67) -> ("latd_ini [º]"=w53:dbl, "lon_ini [º]"=w54:dbl, "alt_ini(m)"=w55:dbl, "V_ini [m/s]"=w66:dbl[], "q ini"=w65:dbl[], w64:dbl[], "W ini [rad/s]"=w63:dbl[], "acc"=w62:dbl[], w61:dbl[], w60:dbl[], "TVA_b"=w59:dbl[], "array"=w58:dbl[], "array"=w57:dbl[], "Pdin"=w56:dbl)  [unwired: 1 out]
          }
          frame Enabled {
          }
        }
      }
    }
    frame #2 {
      n129 = case shown="\"Velocity\"" "Tab Control" {
        tunnel: w533 -> [_ _ _ _ _ _ _ _ _ _ w559 _]
        tunnel: w532 -> [_ _ _ _ _ _ _ _ _ w554 _ _]
        tunnel: w531 -> [w545 _ _ _ _ _ _ _ _ _ _ _]
        tunnel: w530 -> [_ w546 _ _ _ _ _ _ _ _ _ _]
        tunnel: w529 -> [_ _ w547 _ _ _ _ _ _ _ _ _]
        tunnel: w528 -> [_ _ _ w548 _ _ _ _ _ _ _ _]
        tunnel: w527 -> [_ _ _ _ w549 _ _ _ _ _ _ _]
        tunnel: w526 -> [_ _ _ _ _ w550 _ _ _ _ _ _]
        tunnel: w525 -> [_ _ _ _ _ _ w551 _ _ _ _ _]
        tunnel: w524 -> [_ _ _ _ _ _ _ w552 _ _ _ _]
        tunnel: w523 -> [_ _ _ _ _ _ _ _ w553 _ _ _]
        tunnel: w522 -> [_ _ _ _ _ _ _ _ _ _ _ w564]
        tunnel: w521 -> [_ _ _ _ _ _ _ _ _ _ _ w563]
        tunnel: w520 -> [_ _ _ _ _ _ _ _ _ _ _ w562]
        frame "Attitude Euler Angles" {
          n130 = expression code="(x/pi)*180.0" "radians to degrees"(w545) -> (w540:dbl[][])
          n131 = Index Array(array=w540, index (col) #1=0 ("index")) -> (element #1=w539:dbl[], element #2=w537:dbl[], element #3=w536:dbl[])  [unwired: 5 in]
          n132 = Build Array(w539, w537, w536) -> (w538:dbl[][])
          n133 = Bundle(0.0, 0.01, w538) -> (→"Euler Angles [º]":cluster{dbl, dbl, dbl[][]})  [unwired: 1 in]
        }
        frame "Body Rates" {
          "Body Rates" <- w546
        }
        frame "Body Accel" {
          "Body accelerations" <- w547
        }
        frame "Malpha/ Mbeta" {
          "Malpha/Mbeta" <- w548
        }
        frame "AoA" {
          "AoA" <- w549
        }
        frame "TVA nozzle angles" {
          "TVA angles" <- w550
        }
        frame "Oil Consumption" {
          "Oil Consumption" <- w551
        }
        frame "Bending Moments" {
          "Bending Moments" <- w552
        }
        frame "Aerodynamic pressure" {
          "Aerodynamic pressure" <- w553
        }
        frame "Attitude Quaternions" {
          "Quaternions" <- w554
        }
        frame "Velocity" {
          n134 = Index Array(array=w559, index (col) #1=0 ("index")) -> (element #1=w555:dbl[])  [unwired: 5 in, 2 out]
          n135 = Bundle(0.0, 0.01, "V_ini [m/s]"=w555) -> (→"Velocity [m/s]":cluster{dbl, dbl, "V_ini [m/s]":dbl[]})  [unwired: 1 in]
          "V_ini [m/s]" <- w559
        }
        frame "Position" {
          n136 = Build Array(w562, w563, w564) -> (→"Position":dbl[][])
        }
      }
      n137 = property on="Run_SIM" class="Bool (strict)"("Value"=FALSE) -> ()  [unwired: 2 in, 2 out]
    }
  }
